vi "Motion-Close.vi"(8 "error in (no error)":errorcluster, 11 "Motion-ControlAll in":refnum<class "Motion-ControlAll.lvclass">) -> (0 "error out":errorcluster, 3 "Motion-ControlAll out":refnum<class "Motion-ControlAll.lvclass">)   [LabVIEW 2013, in "Motion-ControlAll.lvclass"]
uses:
  Motion-ControlAll.lvclass
  Motion-ControlAll.lvclass/Motion-ControlAll.ctl
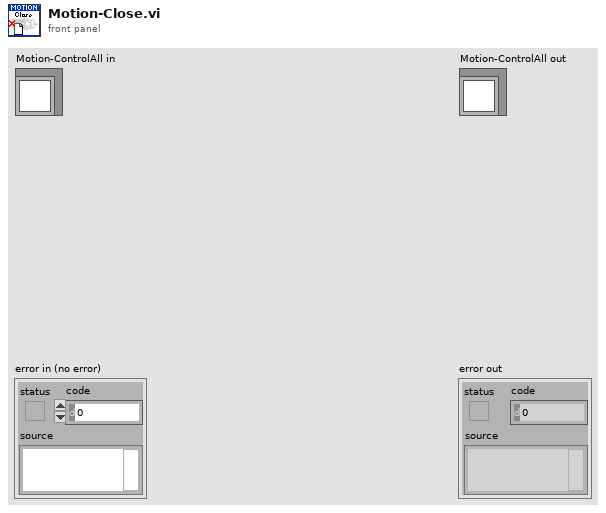
[diagram p1: front panel]
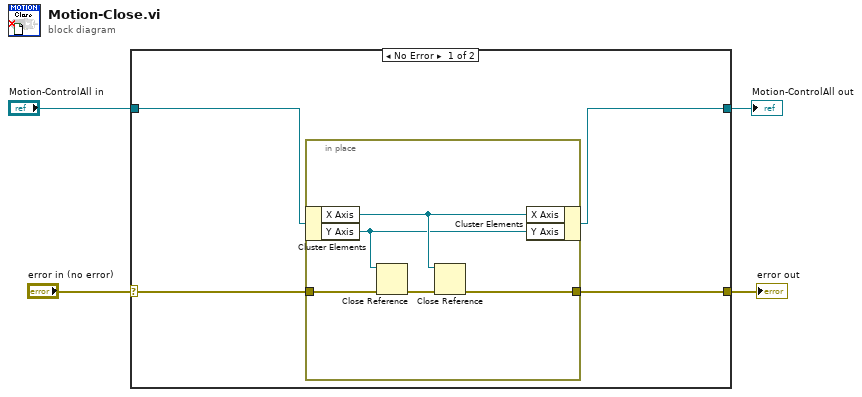
[diagram p0: block diagram]
diagram:
  n1 = case shown="No Error" "error in (no error)" {
    selector: "error in (no error)" -> [w7 w15]
    tunnel: [w6 w15] -> w3
    tunnel: [w5 w14] -> w1
    tunnel: "Motion-ControlAll in" -> [w8 w14]
    frame No Error {
      n2 = in-place {
        in-place-border: w7 -> [w13]
        in-place-border: [w9] -> w6
        n3 = in-place-cluster #1(w8) -> ("X Axis"=w11:refnum<k7>, "Y Axis"=w10:refnum<k7>)
        n4 = Close Reference(reference=w10, error in (no error)=w13) -> (error out=w12:errorcluster)
        n5 = Close Reference(reference=w11, error in (no error)=w12) -> (error out=w9:errorcluster)
        n6 = in-place-cluster #1("X Axis"=w11, "Y Axis"=w10) -> (w5:refnum<class "Motion-ControlAll.lvclass">)
      }
    }
    frame Error {
    }
  }
  "error out" <- w3
  "Motion-ControlAll out" <- w1
